vi "Read New Card Ref.vi"(8 "error in (no error)":errorcluster, 11 "Generic Instrument in":refnum<class "Generic Instrument.lvclass">) -> (0 "error out":errorcluster, 2 "New Card Ref":refnum<vi>, 3 "Generic Instrument out":refnum<class "Generic Instrument.lvclass">)   [LabVIEW 2016, in "Generic Instrument.lvlib" / "Generic Instrument.lvclass"]
uses:
  Generic Instrument.lvclass
  Generic Instrument.lvclass/Generic Instrument.ctl
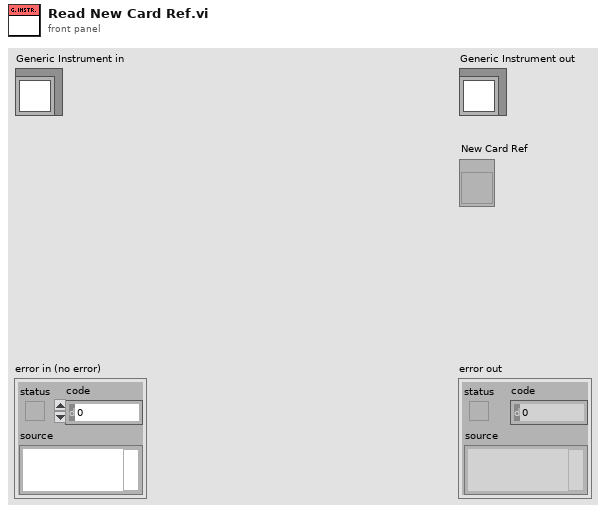
[diagram p1: front panel]
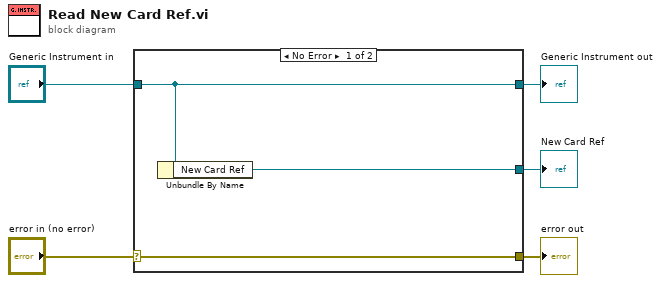
[diagram p0: block diagram]
diagram:
  n1 = case shown="No Error" "error in (no error)" {
    selector: "error in (no error)" -> [w8 w9]
    tunnel: [w8 w9] -> w4
    tunnel: [w7 w10] -> w2
    tunnel: "Generic Instrument in" -> [w7 w10]
    tunnel: [w6 _] -> w1
    frame No Error {
      n2 = Unbundle By Name(w7) -> ("New Card Ref"=w6:refnum<vi>)
    }
    frame Error {
    }
  }
  "error out" <- w4
  "Generic Instrument out" <- w2
  "New Card Ref" <- w1
